vi "Format OBW.vi"(10 "OBW":T2) -> (2 "OBW Results":T1 {"Stop Frequency (Hz)" format="%#_4p"; "Start Frequency (Hz)" format="%#_4p"})   [LabVIEW 2015, in "niDTS BT.lvlib" / "niDTS BT INSTR TX.lvclass"]
uses:
  niDTS BT INSTR TX.lvclass
  Tests/Tx Test/Includes/niDTS BT Tx Test INC OBW Results.ctl
  niDTS BT.lvlib
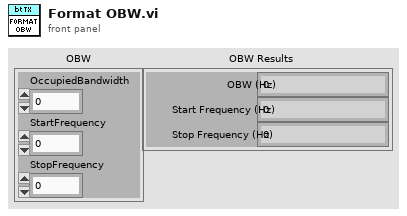
[diagram p1: front panel]
types:
  T1 = typedef "niDTS BT.lvlib/niDTS BT Tx Test INC OBW Results.ctl" = cluster{"OBW (Hz)":dbl, "Start Frequency (Hz)":dbl, "Stop Frequency (Hz)":dbl}
  T2 = cluster{"OccupiedBandwidth":dbl, "StartFrequency":dbl, "StopFrequency":dbl}
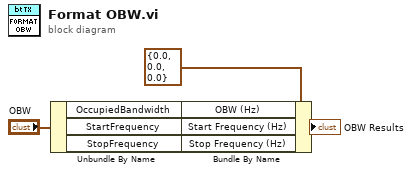
[diagram p0: block diagram]
diagram:
  n1 = Unbundle By Name("OBW") -> ("OccupiedBandwidth"=w4:dbl, "StartFrequency"=w3:dbl, "StopFrequency"=w2:dbl)
  n2 = Bundle By Name(cluster=T1 {"OBW (Hz)"=0.0, "Start Frequency (Hz)"=0.0, "Stop Frequency (Hz)"=0.0} ("OBW Resutls"), "OBW (Hz)"=w4, "Start Frequency (Hz)"=w3, "Stop Frequency (Hz)"=w2) -> (→"OBW Results":T1)
